vi "Create Tag Channel Pair.vi"(10 "Tag Name":string, 11 "Channel Name":string) -> (3 "tag channel pair":T1)   [LabVIEW 2013, in "Engine Runtime Interface.lvclass"]
uses:
  Engine Runtime Interface.lvclass
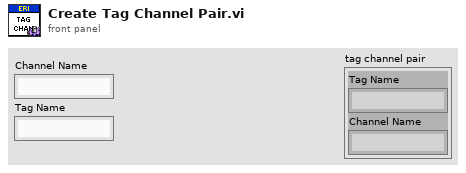
[diagram p1: front panel]
types:
  T1 = cluster{"Tag Name":string, "Channel Name":string}
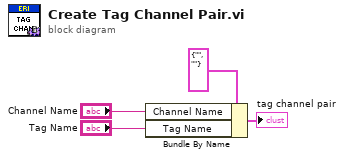
[diagram p0: block diagram]
diagram:
  n1 = Bundle By Name(cluster=T1 {"Tag Name"="", "Channel Name"=""} ("Mapping"), "Channel Name"="Channel Name", "Tag Name"="Tag Name") -> (→"tag channel pair":T1)
